vi "Init Environment.vi"(8 "error in (no error)":errorcluster, 11 "Test Framework in":refnum<class "Test Framework.lvclass">) -> (0 "error out":errorcluster, 3 "Test Framework out":refnum<class "Test Framework.lvclass">)   [LabVIEW 2020, in "Test Framework.lvclass"]
uses:
  Test Framework.lvclass
  Controls/Temperature and voltage modes.ctl
  Test Framework.lvclass/Test Framework.ctl
  Instruments/Temperature Control/Temperature Control.lvclass
  Instruments/Temperature Control/Controls/Head and Air actions.ctl
  Instruments/Power Supply/Power Supply.lvclass
  C:/Sandbox/Git_Sandbox/WiSpry Test Framework source code (LV20)/WiSpry Test Framework/Instruments/Instrument.lvclass
  Instruments/Power Supply/Controls/Source mode.ctl
  Instruments/Instrument.lvclass/Instrument.ctl
  Instruments/Power Supply/Power Supply.lvclass/Power Supply.ctl
  Instruments/Instrument.lvclass
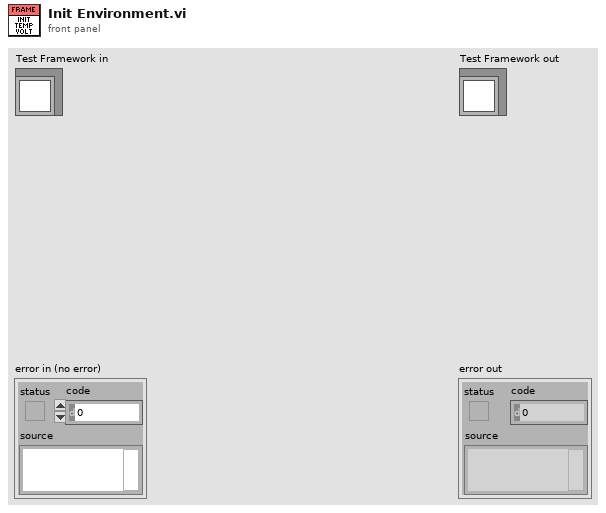
[diagram p1: front panel]
types:
  T1 = enum16{"Temperature Mode", "Init Temperature Control", "Init PSU", "Done"}
  T2 = typedef "Test Framework.lvclass/Temperature and voltage modes.ctl" = cluster{"Temperature mode":enum16{"Automatic", "Manual", "Off"}, "DC-Power mode":enum16{"Automatic", "Manual", "Off"}, "PSU sweep mode":bool, "Turn off after measurement":bool}
  T3 = typedef "Temperature Control.lvclass/Head and Air actions.ctl" = enum16{"Head Down & Air On", "Head Up & Air Off", "Head Down", "Head Up", "Air On", "Air Off", "Compressor On", "Compressor Off"}
  T4 = cluster{"Number":u32, "Temperature":dbl, "Temperature Window":dbl, "Soak Time [s]":u32, "Ramp Rate":dbl}
  T5 = typedef "Power Supply.lvclass/Source mode.ctl" = enum32{"Voltage", "Current"}
  T6 = typedef "Test Framework.lvclass/Temperature and voltage array.ctl" = cluster{"Temperature [C]":dbl, "Soak time [m]":dbl, "PSUs":cluster{"Enabled":bool, "Source":enum32{"Voltage", "Current"}, "Drive (V/A)":dbl, "Sweep (V/A)":string, "Limit (A/V)":dbl, "PSU alias":string, "PSU info":cluster{"ID":string, "Address":string, "Channel":u8}}[]}[]
  T7 = cluster{"Temperature control array":T6, "Temperature mode":T2}
  T8 = cluster{"Instrument Name":string, "Instrument.lvclass":refnum<class "Instrument.lvclass">, "Reference":bool}[]
  T9 = cluster{"Temperature [C]":dbl, "Soak time [m]":dbl, "PSUs":cluster{"Enabled":bool, "Source":enum32{"Voltage", "Current"}, "Drive (V/A)":dbl, "Sweep (V/A)":string, "Limit (A/V)":dbl, "PSU alias":string, "PSU info":cluster{"ID":string, "Address":string, "Channel":u8}}[]}
  T10 = cluster{"Enabled":bool, "Source":enum32{"Voltage", "Current"}, "Drive (V/A)":dbl, "Sweep (V/A)":string, "Limit (A/V)":dbl, "PSU alias":string, "PSU info":cluster{"ID":string, "Address":string, "Channel":u8}}[]
  T11 = typedef "Instrument.lvclass/Interface String Cluster.ctl" = cluster{"Interface":string, "IDN string":string, "Instance":i32}
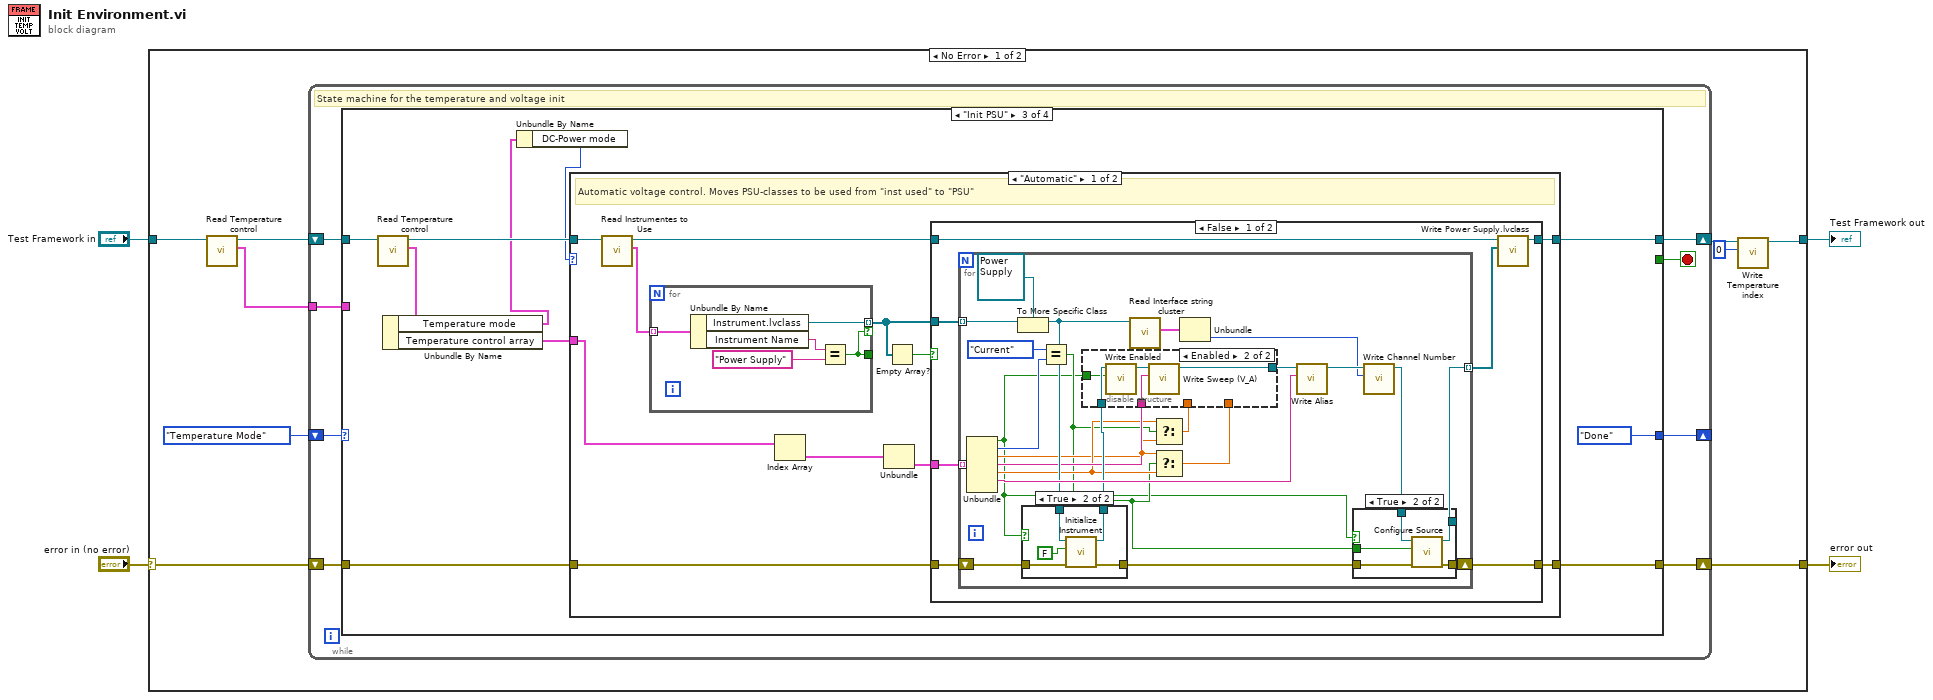
[diagram p0: block diagram]
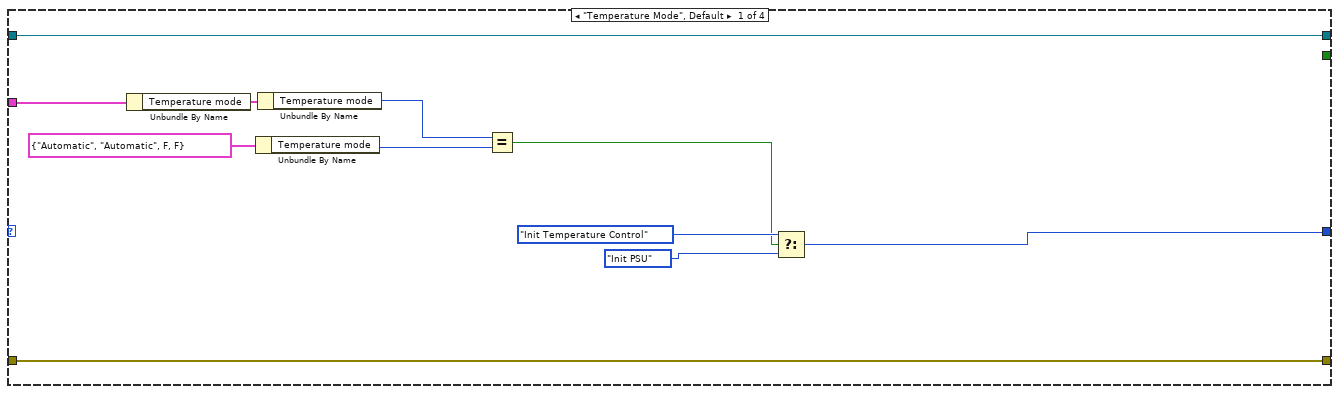
[diagram p2: hidden frame]
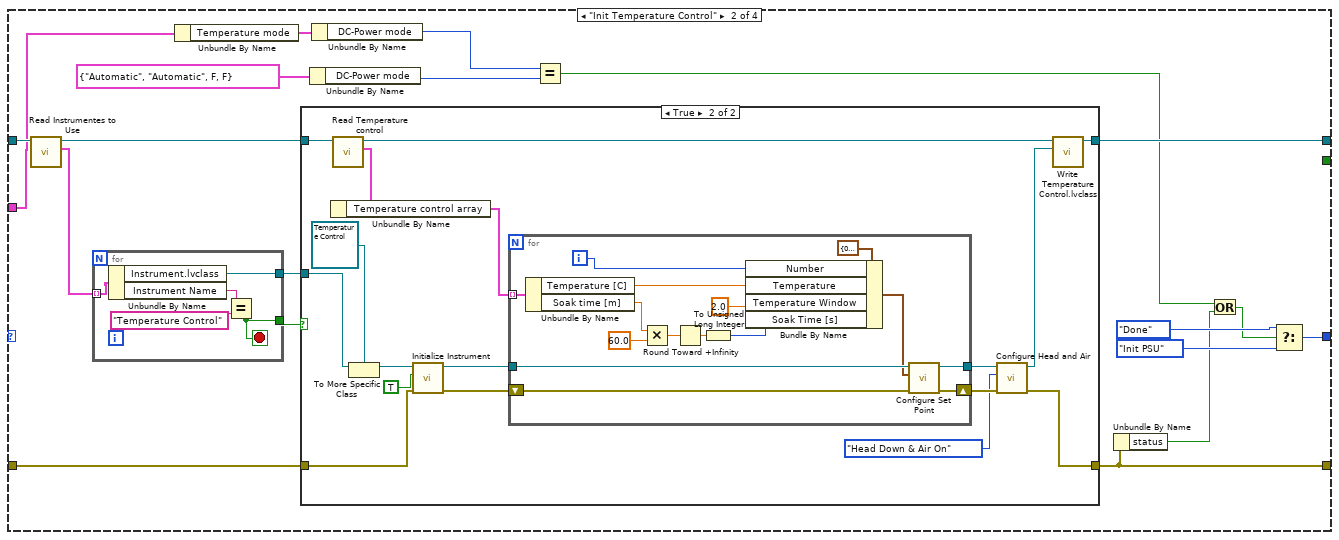
[diagram p3: hidden frame]
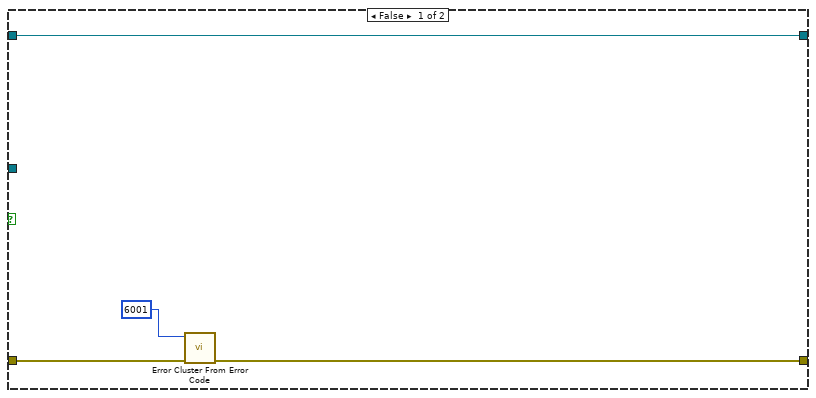
[diagram p4: hidden frame]
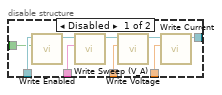
[diagram p6: hidden frame]
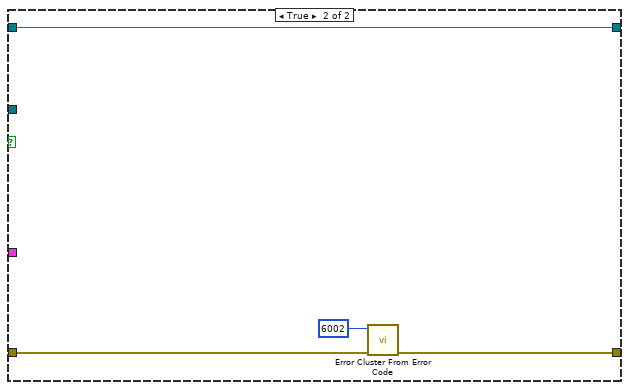
[diagram p8: hidden frame]
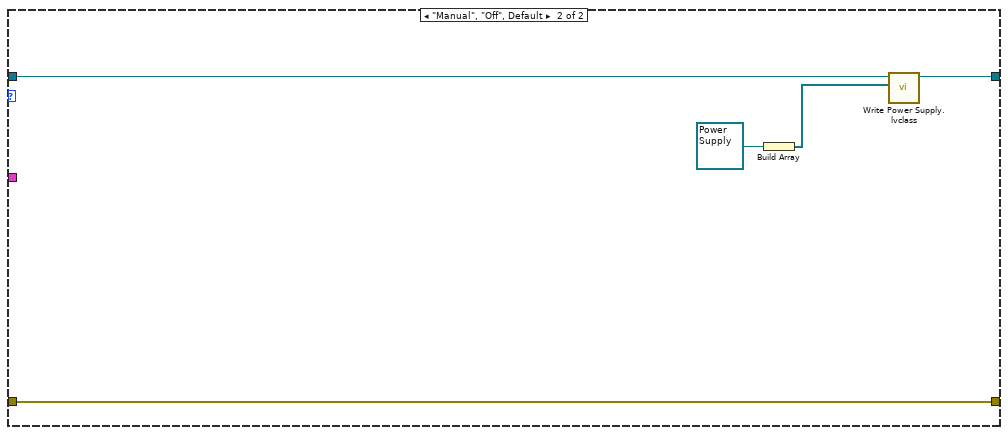
[diagram p9: hidden frame]
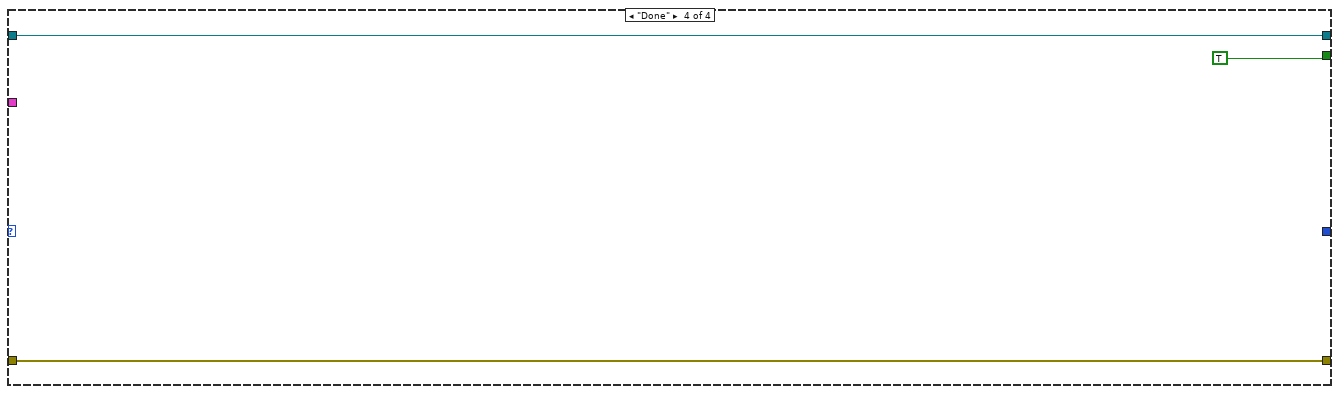
[diagram p10: hidden frame]
diagram:
  n1 = case shown="No Error" "error in (no error)" {
    selector: "error in (no error)" -> [w13 w191]
    tunnel: [w11 w191] -> w3
    tunnel: [w9 w190] -> w1
    tunnel: "Test Framework in" -> [w7 w190]
    frame No Error {
      n2 = call-dynamic "Read Temperature control.vi"("Test Framework in"=w7) -> ("Temperature control"=w5:T7, "Test Framework out"=w6:refnum<class "Test Framework.lvclass">)  [unwired: 9 in]
      n3 = while {
        shift-right: [w16] -> w11
        shift-left: w13 -> [w20]
        shift-right: [w17] -> _
        shift-left: T1."Temperature Mode" -> [w19]
        shift-right: [w18] -> w10
        shift-left: w6 -> [w21]
        tunnel: w5 -> [w14]
        stop <- w15 stop-if-true
        # "State machine for the temperature and voltage init"
        n4 = case shown="\"Init PSU\"" w19 {
          tunnel: w21 -> [w27 w51 w102 w188]
          tunnel: w20 -> [w29 w45 w99 w187]
          tunnel: [w27 w46 w97 w188] -> w18
          tunnel: [w31 w44 T1."Done" ("f") _] -> w17
          tunnel: [w29 w36 w98 w187] -> w16
          tunnel: [_ _ _ TRUE] -> w15
          tunnel: w14 -> [w28 w37 _ _]
          frame "Temperature Mode", Default {
            n5 = Unbundle By Name(w28) -> ("Temperature mode"=w26:T2)
            n6 = Unbundle By Name(T2 {"Temperature mode"=enum."Automatic", "DC-Power mode"=enum."Automatic", "PSU sweep mode"=FALSE, "Turn off after measurement"=FALSE} ("Temperature mode")) -> ("Temperature mode"=w24:enum16{"Automatic", "Manual", "Off"})
            n7 = Unbundle By Name(w26) -> ("Temperature mode"=w25:enum16{"Automatic", "Manual", "Off"})
            n8 = Equal?(x=w25, y=w24) -> (x = y?=w22:bool)
            n9 = Select(t=T1."Init Temperature Control", s=w22, f=T1."Init PSU") -> (s? t:f=w31:T1)
          }
          frame "Init Temperature Control" {
            n10 = call "Read Instrumentes to Use.vi"("Test Framework in"=w51) -> ("Instrumentes to Use"=w50:T8, "Test Framework out"=w47:refnum<class "Test Framework.lvclass">)  [unwired: 9 in]
            n11 = for {
              tunnel: w50 -> [w92] mode=indexing
              tunnel: [w89] -> w48
              tunnel: [w88] -> w49
              stop <- w88 stop-if-true
              n12 = Unbundle By Name(w92) -> ("Instrument.lvclass"=w89:refnum<class "Instrument.lvclass">, "Instrument Name"=w91:string)
              n13 = Equal?(x=w91, y="Temperature Control") -> (x = y?=w88:bool)
            }
            n14 = Unbundle By Name(w37) -> ("Temperature mode"=w41:T2)
            n15 = case shown="True" w49 {
              tunnel: w48 -> [_ w72]
              tunnel: w47 -> [w55 w67]
              tunnel: [w55 w68] -> w46
              tunnel: [w53 w57] -> w36
              tunnel: w45 -> [w54 w61]
              frame False {
                n16 = call <vilib>:"Error Cluster From Error Code.vi"("error in (no error)"=w54, "error code (0)"=6001 ("Error Code")) -> ("error out"=w53:errorcluster)  [unwired: 7 in]
              }
              frame True {
                n17 = call-dynamic "Read Temperature control.vi"("Test Framework in"=w67) -> ("Temperature control"=w65:T7, "Test Framework out"=w66:refnum<class "Test Framework.lvclass">)  [unwired: 9 in]
                n18 = Unbundle By Name(w65) -> ("Temperature control array"=w64:T6)
                n19 = To More Specific Class(target class=refnum<class "Temperature Control.lvclass"> refnum ("Temperature Control.lvclass"), reference=w72) -> (specific class reference=w70:refnum<class "Temperature Control.lvclass">)  [unwired: 1 in, 1 out]
                n20 = call-dynamic "Initialize Instrument.vi"("error in (no error)"=w61, "Reset"=TRUE, "Instrument in"=w70) -> ("error out"=w62:errorcluster, "Instrument out"=w63:refnum<class "Temperature Control.lvclass">)  [unwired: 7 in]
                n21 = for {
                  tunnel: w64 -> [w84] mode=indexing
                  tunnel: w63 -> [w87]
                  tunnel: [w75] -> w60
                  shift-right: [w73] -> w58
                  shift-left: w62 -> [w74]
                  i -> [w85]
                  n22 = Unbundle By Name(w84) -> ("Temperature [C]"=w83:dbl, "Soak time [m]"=w82:dbl)
                  n23 = Multiply(x=w82, y=60.0) -> (x*y=w79:dbl)
                  n24 = Round Toward +Infinity(x=w79) -> (ceil(x): smallest int >= x=w78:dbl)
                  n25 = To Unsigned Long Integer(number=w78) -> (unsigned 32bit integer=w77:u32)
                  n26 = Bundle By Name(cluster=T4 {"Number"=0, "Temperature"=0.0, "Temperature Window"=0.0, "Soak Time [s]"=0, "Ramp Rate"=0.0} ("Set Point"), "Number"=w85, "Temperature"=w83, "Temperature Window"=2.0, "Soak Time [s]"=w77) -> (w76:T4)
                  n27 = call-dynamic "Configure Set Point.vi"("error in (no error)"=w74, "Set Point"=w76, "Temperature Control in"=w87) -> ("error out"=w73:errorcluster, "Temperature Control out"=w75:refnum<class "Temperature Control.lvclass">)  [unwired: 7 in]
                }
                n28 = call-dynamic "Configure Head and Air.vi"("error in (no error)"=w58, "Head and Air actions"=Head_and_Air_actions."Head Down & Air On", "Temperature Control in"=w60) -> ("error out"=w57:errorcluster, "Temperature Control out"=w59:refnum<class "Temperature Control.lvclass">)  [unwired: 7 in]
                n29 = call "Write Temperature Control.lvclass.vi"("Temperature Control.lvclass"=w59, "Test Framework in"=w66) -> ("Test Framework out"=w68:refnum<class "Test Framework.lvclass">)  [unwired: 9 in]
              }
            }
            n30 = Unbundle By Name(T2 {"Temperature mode"=enum."Automatic", "DC-Power mode"=enum."Automatic", "PSU sweep mode"=FALSE, "Turn off after measurement"=FALSE} ("Temperature mode")) -> ("DC-Power mode"=w39:enum16{"Automatic", "Manual", "Off"})
            n31 = Unbundle By Name(w41) -> ("DC-Power mode"=w40:enum16{"Automatic", "Manual", "Off"})
            n32 = Equal?(x=w40, y=w39) -> (x = y?=w34:bool)
            n33 = Unbundle By Name(w36) -> ("status"=w35:bool)
            n34 = Or(x=w34, y=w35) -> (x .or. y?=w33:bool)
            n35 = Select(t=T1."Done", s=w33, f=T1."Init PSU") -> (s? t:f=w44:T1)
          }
          frame "Init PSU" {
            n36 = call-dynamic "Read Temperature control.vi"("Test Framework in"=w102) -> ("Temperature control"=w101:T7, "Test Framework out"=w100:refnum<class "Test Framework.lvclass">)  [unwired: 9 in]
            n37 = Unbundle By Name(w101) -> ("Temperature mode"=w94:T2, "Temperature control array"=w95:T6)
            n38 = Unbundle By Name(w94) -> ("DC-Power mode"=w93:enum16{"Automatic", "Manual", "Off"})
            n39 = case shown="\"Automatic\"" w93 {
              tunnel: w100 -> [w113 w185]
              tunnel: w99 -> [w110 w184]
              tunnel: [w109 w184] -> w98
              tunnel: [w108 w186] -> w97
              tunnel: w95 -> [w105 _]
              frame "Automatic" {
                # "Automatic voltage control. Moves PSU-classes to be used from \"inst used\" to \"PSU\""
                n40 = call "Read Instrumentes to Use.vi"("Test Framework in"=w113) -> ("Instrumentes to Use"=w112:T8, "Test Framework out"=w111:refnum<class "Test Framework.lvclass">)  [unwired: 9 in]
                n41 = for {
                  tunnel: w112 -> [w181] mode=indexing
                  tunnel: [w178] -> w106 mode=indexing if=w177
                  tunnel: [w177] -> _
                  n42 = Unbundle By Name(w181) -> ("Instrument.lvclass"=w178:refnum<class "Instrument.lvclass">, "Instrument Name"=w180:string)
                  n43 = Equal?(x=w180, y="Power Supply") -> (x = y?=w177:bool)
                }
                n44 = Index Array(array=w105) -> (element=w104:T9)  [unwired: 1 in]
                n45 = Unbundle(w104) -> ("PSUs"=w103:T10)  [unwired: 2 out]
                n46 = Empty Array?(array=w106) -> (empty?=w107:bool)
                n47 = case shown="False" w107 {
                  tunnel: w111 -> [w115 w176]
                  tunnel: w106 -> [w120 _]
                  tunnel: w110 -> [w119 w174]
                  tunnel: [w117 w175] -> w109
                  tunnel: [w118 w176] -> w108
                  tunnel: w103 -> [w114 _]
                  frame False {
                    n48 = for {
                      tunnel: w120 -> [w144] mode=indexing
                      tunnel: [w125] -> w116 mode=indexing
                      shift-right: [w126] -> w117
                      shift-left: w119 -> [w142]
                      tunnel: w114 -> [w140] mode=indexing
                      n49 = Unbundle(w140) -> ("Enabled"=w121:bool, "Source"=w139:enum32{"Voltage", "Current"}, "Drive (V/A)"=w128:dbl, "Sweep (V/A)"=w132:string, "Limit (A/V)"=w129:dbl, "PSU alias"=w138:string)  [unwired: 1 out]
                      n50 = To More Specific Class(target class=refnum<class "Power Supply.lvclass"> refnum ("Power Supply.lvclass"), reference=w144) -> (specific class reference=w136:refnum<class "Power Supply.lvclass">)  [unwired: 1 in, 1 out]
                      n51 = case shown="True" w121 {
                        tunnel: w142 -> [w167 w172]
                        tunnel: [w167 w171] -> w127
                        tunnel: w136 -> [w166 w169]
                        tunnel: [w166 w168] -> w133
                        frame False {
                        }
                        frame True {
                          n52 = call-dynamic "Initialize Instrument.vi"("error in (no error)"=w172, "Reset"=FALSE, "Power Supply in"=w169) -> ("error out"=w171:errorcluster, "Power Supply out"=w168:refnum<class "Power Supply.lvclass">)  [unwired: 7 in]
                        }
                      }
                      n53 = Equal?(x=Source_mode."Current" ("Source"), y=w139) -> (x = y?=w122:bool)
                      n54 = call "Read Interface string cluster.vi"("Instrument in"=w136) -> ("Interface sting cluster"=w135:T11)  [unwired: 9 in, 1 out]
                      n55 = Select(t=w129, s=w122, f=w128) -> (s? t:f=w130:dbl)
                      n56 = Select(t=w128, s=w122, f=w129) -> (s? t:f=w131:dbl)
                      n57 = disable-structure shown="Enabled" {
                        disable-tunnel: w133 -> [w160 w162]
                        disable-tunnel: w132 -> [w156 w164]
                        disable-tunnel: w131 -> [w155 _]
                        disable-tunnel: w130 -> [w154 _]
                        disable-tunnel: w121 -> [w153 w161]
                        disable-tunnel: [w152 w165] -> w123
                        frame Disabled {
                          n58 = call-dynamic "Write Enabled.vi"("Enabled"=w153, "Power Supply in"=w160) -> ("Power Supply out"=w159:refnum<class "Power Supply.lvclass">)  [unwired: 9 in]
                          n59 = call-dynamic "Write Sweep (V_A).vi"("Sweep (V/A)"=w156, "Power Supply in"=w159) -> ("Power Supply out"=w158:refnum<class "Power Supply.lvclass">)  [unwired: 9 in]
                          n60 = call "Write Voltage.vi"("Voltage"=w154, "Power Supply in"=w158) -> ("Power Supply out"=w157:refnum<class "Power Supply.lvclass">)  [unwired: 9 in]
                          n61 = call "Write Current.vi"("Current"=w155, "Power Supply in"=w157) -> ("Power Supply out"=w152:refnum<class "Power Supply.lvclass">)  [unwired: 9 in]
                        }
                        frame Enabled {
                          n62 = call-dynamic "Write Enabled.vi"("Enabled"=w161, "Power Supply in"=w162) -> ("Power Supply out"=w163:refnum<class "Power Supply.lvclass">)  [unwired: 9 in]
                          n63 = call-dynamic "Write Sweep (V_A).vi"("Sweep (V/A)"=w164, "Power Supply in"=w163) -> ("Power Supply out"=w165:refnum<class "Power Supply.lvclass">)  [unwired: 9 in]
                        }
                      }
                      n64 = Unbundle(w135) -> ("Instance"=w134:i32)  [unwired: 2 out]
                      n65 = call-dynamic "Write Alias.vi"("Alias"=w138, "Power Supply in"=w123) -> ("Power Supply out"=w137:refnum<class "Power Supply.lvclass">)  [unwired: 9 in]
                      n66 = call "Write Channel Number.vi"("Channel Number"=w134, "Power Supply in"=w137) -> ("Power Supply out"=w124:refnum<class "Power Supply.lvclass">)  [unwired: 9 in]
                      n67 = case shown="True" w121 {
                        tunnel: w127 -> [w145 w151]
                        tunnel: [w145 w150] -> w126
                        tunnel: [w146 w149] -> w125
                        tunnel: w124 -> [w146 w148]
                        tunnel: w122 -> [_ w147]
                        frame False {
                        }
                        frame True {
                          n68 = call-dynamic "Configure Source.vi"("error in (no error)"=w151, "Source (F:Volt)"=w147, "Power Supply in"=w148) -> ("error out"=w150:errorcluster, "Power Supply out"=w149:refnum<class "Power Supply.lvclass">)  [unwired: 7 in]
                        }
                      }
                    }
                    n69 = call "Write Power Supply.lvclass.vi"("Power Supply lvclasses"=w116, "Test Framework in"=w115) -> ("Test Framework out"=w118:refnum<class "Test Framework.lvclass">)  [unwired: 9 in]
                  }
                  frame True {
                    n70 = call <vilib>:"Error Cluster From Error Code.vi"("error in (no error)"=w174, "error code (0)"=6002 ("Error Code")) -> ("error out"=w175:errorcluster)  [unwired: 7 in]
                  }
                }
              }
              frame "Manual", "Off", Default {
                n71 = Build Array(refnum<class "Power Supply.lvclass"> refnum ("Power Supply.lvclass")) -> (w182:refnum<class "Power Supply.lvclass">[])
                n72 = call "Write Power Supply.lvclass.vi"("Power Supply lvclasses"=w182, "Test Framework in"=w185) -> ("Test Framework out"=w186:refnum<class "Test Framework.lvclass">)  [unwired: 9 in]
              }
            }
          }
          frame "Done" {
          }
        }
      }
      n73 = call "Write Temperature index.vi"("Environmental index"=0 ("Temperature index"), "Test Framework in"=w10) -> ("Test Framework out"=w9:refnum<class "Test Framework.lvclass">)  [unwired: 9 in]
    }
    frame Error {
    }
  }
  "error out" <- w3
  "Test Framework out" <- w1
